vi "HeaderRe-Arrange.vi"(8 "error in (no error)":errorcluster, 9 "Data in":string, 10 "New Header":string[](array[string]), 11 "Old DataCluster":string) -> (0 "error out":errorcluster, 2 "Data Out":string, 3 "Results":string)   [LabVIEW 2014, in "TableLogger_CSV_Actor.lvlib" / "TableLogger_CSV_Actor.lvclass"]
uses:
  TableLogger_CSV_Actor.lvclass
  <userlib>/_OpenG.lib/array/array.llb/Remove Duplicates from 1D Array (String)__ogtk.vi
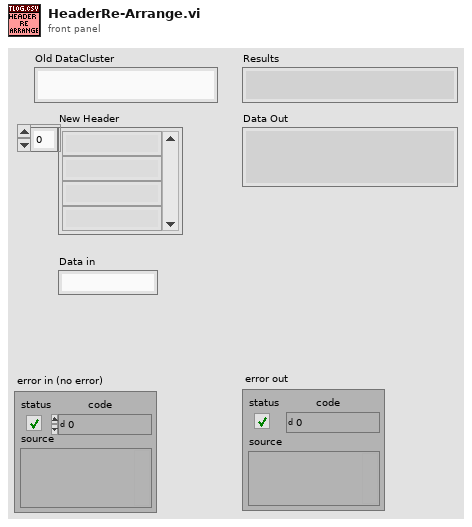
[diagram p1: front panel]
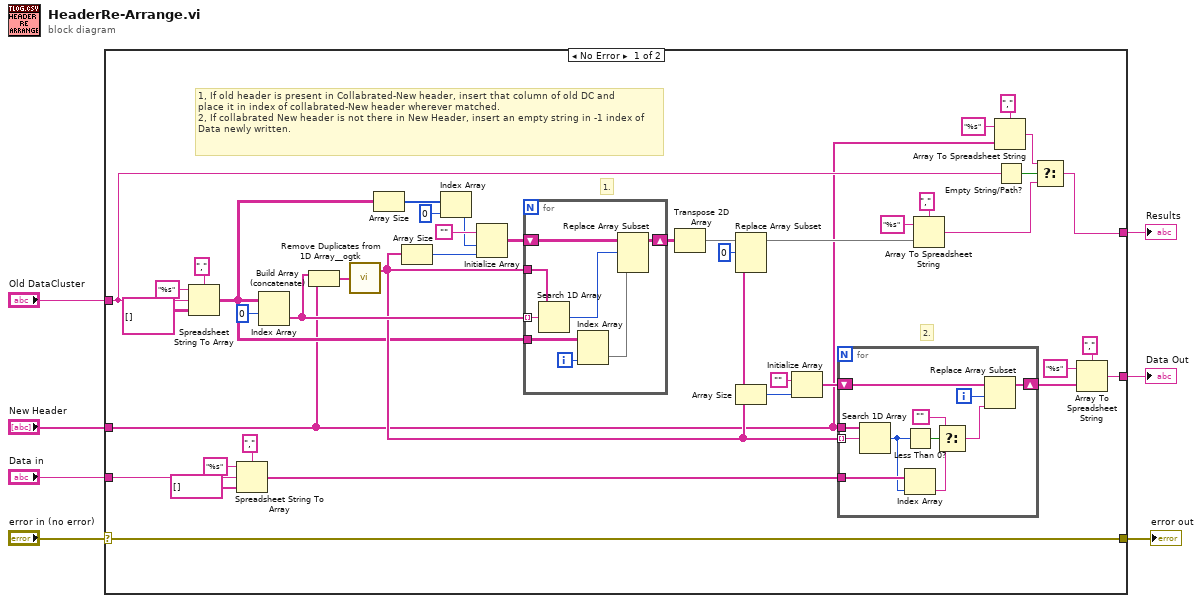
[diagram p0: block diagram]
diagram:
  n1 = case shown="No Error" "error in (no error)" {
    selector: "error in (no error)" -> [w21 w68]
    tunnel: "Data in" -> [w17 w69]
    tunnel: "Old DataCluster" -> [w15 w70]
    tunnel: [w8 w70] -> w5
    tunnel: [w32 w69] -> w7
    tunnel: "New Header" -> [w11 _]
    tunnel: [w21 w68] -> w2
    frame No Error {
      # "2."
      # "1."
      # "1, If old header is present in Collabrated-New header, insert that column of old DC and\nplace it in index of collabrated-New header wherever matched.\n2, If collabrated New header is not there in New Header, insert an empty string in -1 index of Data newly written."
      n2 = Spreadsheet String To Array(delimiter (Tab)=",", format string="%s", spreadsheet string=w15, array type (2D Dbl)=string[][] [] ("output array")) -> (array=w24:string[][])
      n3 = Spreadsheet String To Array(delimiter (Tab)=",", format string="%s", spreadsheet string=w17, array type (2D Dbl)=string[] [] ("output array")) -> (array=w16:string[])
      n4 = Index Array(array=w24, index (row)=0) -> (element=w30:string[])  [unwired: 1 in]
      n5 = Build Array (concatenate)(w30, w11) -> (w31:string[])
      n6 = call-poly <userlib>:"Remove Duplicates from 1D Array__ogtk.vi"("Input Array"=w31) -> ("Output Array"=w29:string[])  [unwired: 1 out]
      n7 = Array Size(array=w24) -> (size(s)=w44:i32[])
      n8 = Array Size(array=w29) -> (size(s)=w45:i32)
      n9 = Index Array(array=w44, index=0) -> (element=w43:i32)
      n10 = Initialize Array("", w43, w45) -> (w42:string[][])
      n11 = for {
        tunnel: w29 -> [w66]
        tunnel: w30 -> [w67] mode=indexing
        tunnel: w24 -> [w65]
        shift-right: [w60] -> w48
        shift-left: w42 -> [w63]
        i -> [w64]
        n12 = Search 1D Array(1D array=w66, element=w67) -> (index of element=w62:i32)  [unwired: 1 in]
        n13 = Index Array(array=w65, index (col)=w64) -> (element=w61:string[])  [unwired: 1 in]
        n14 = Replace Array Subset(array=w63, new element=w61, index (row)=w62) -> (w60:string[][])  [unwired: 1 in]
      }
      n15 = Transpose 2D Array(2D array=w48) -> (transposed array=w41:string[][])
      n16 = Replace Array Subset(array=w41, new element=w29, index (row)=0) -> (w26:string[][])  [unwired: 1 in]
      n17 = Array Size(array=w29) -> (size(s)=w38:i32)
      n18 = Initialize Array("", w38) -> (w37:string[])
      n19 = for {
        tunnel: w29 -> [w59] mode=indexing
        tunnel: w11 -> [w58]
        shift-right: [w57] -> w35
        shift-left: w37 -> [w56]
        tunnel: w16 -> [w52]
        i -> [w50]
        n20 = Search 1D Array(1D array=w58, element=w59) -> (index of element=w49:i32)  [unwired: 1 in]
        n21 = Less Than 0?(x=w49) -> (x < 0?=w55:bool)
        n22 = Index Array(array=w52, index=w49) -> (element=w51:string)
        n23 = Select(t="", s=w55, f=w51) -> (s? t:f=w54:string)
        n24 = Replace Array Subset(array=w56, new element=w54, index=w50) -> (w57:string[])
      }
      n25 = Array To Spreadsheet String(delimiter (Tab)=",", array=w26, 3:"%s" ("format string")) -> (spreadsheet string=w9:string)
      n26 = Array To Spreadsheet String(delimiter (Tab)=",", array=w11, 3:"%s" ("format string")) -> (spreadsheet string=w10:string)
      n27 = Empty String/Path?(string/path=w15) -> (empty?=w14:bool)
      n28 = Select(t=w10, s=w14, f=w9) -> (s? t:f=w8:string)
      n29 = Array To Spreadsheet String(delimiter (Tab)=",", array=w35, 3:"%s" ("format string")) -> (spreadsheet string=w32:string)
    }
    frame Error {
    }
  }
  "Data Out" <- w7
  "Results" <- w5
  "error out" <- w2
